vi "mb Convert [SGL] to [U16].vi"(4 "SGL":sgl, 5 "SGL [ ]":sgl[](array[numeric])) -> (1 "U16 [ ]":u16[](array[numeric]))   [LabVIEW 2009]
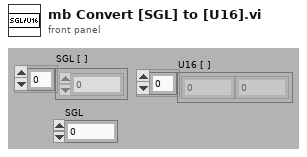
[diagram p1: front panel]
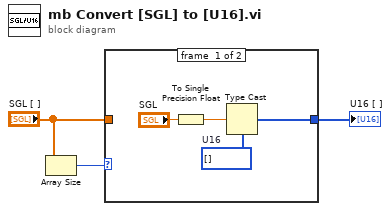
[diagram p0: block diagram]
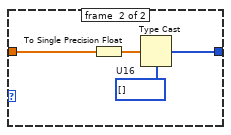
[diagram p2: hidden frame]
diagram:
  n1 = Array Size(array="SGL [ ]") -> (size(s)=w2:i32)
  n2 = case shown="0" w2 {
    tunnel: "SGL [ ]" -> [_ w11]
    tunnel: [w4 w8] -> w1
    frame #0 {
      w6 = u16[] []  # U16
      n3 = To Single Precision Float(number="SGL") -> (single precision float=w7:sgl)
      n4 = Type Cast(type=w6, x=w7) -> (*(type *) &x=w4:u16[])
    }
    frame #1 {
      w9 = u16[] []  # U16
      n5 = To Single Precision Float(number=w11) -> (single precision float=w10:sgl[])
      n6 = Type Cast(type=w9, x=w10) -> (*(type *) &x=w8:u16[])
    }
  }
  "U16 [ ]" <- w1
